vi "DisplayImagePlot.vi"(7 "Data Array":dbl[][](array[numeric]), 8 "Picture For Size Ref":refnum<vi>, 9 "Colormap":bool, 10 "Axis":bool, 11 "Map":T1) -> (2 "Picture":picture)   [LabVIEW 2018]
uses:
  <vilib>/Heliosphere Research LLC/Advanced Plotting Toolkit/properties/Colormap_Map.ctl
  <vilib>/Heliosphere Research LLC/Advanced Plotting Toolkit/api_plotting/ArrayViewProperties.ctl
  <vilib>/Heliosphere Research LLC/Advanced Plotting Toolkit/properties/Colormap.ctl
  <vilib>/Heliosphere Research LLC/Advanced Plotting Toolkit/properties/Colormap_Scaling.ctl
  <vilib>/Heliosphere Research LLC/Advanced Plotting Toolkit/properties/Display.ctl
  <vilib>/Heliosphere Research LLC/Advanced Plotting Toolkit/api_core/NewPlotProperties.ctl
  <vilib>/Heliosphere Research LLC/Advanced Plotting Toolkit/typedefs/PlotColor.ctl
  <vilib>/Heliosphere Research LLC/Advanced Plotting Toolkit/Advanced Plotting Toolkit.lvlib
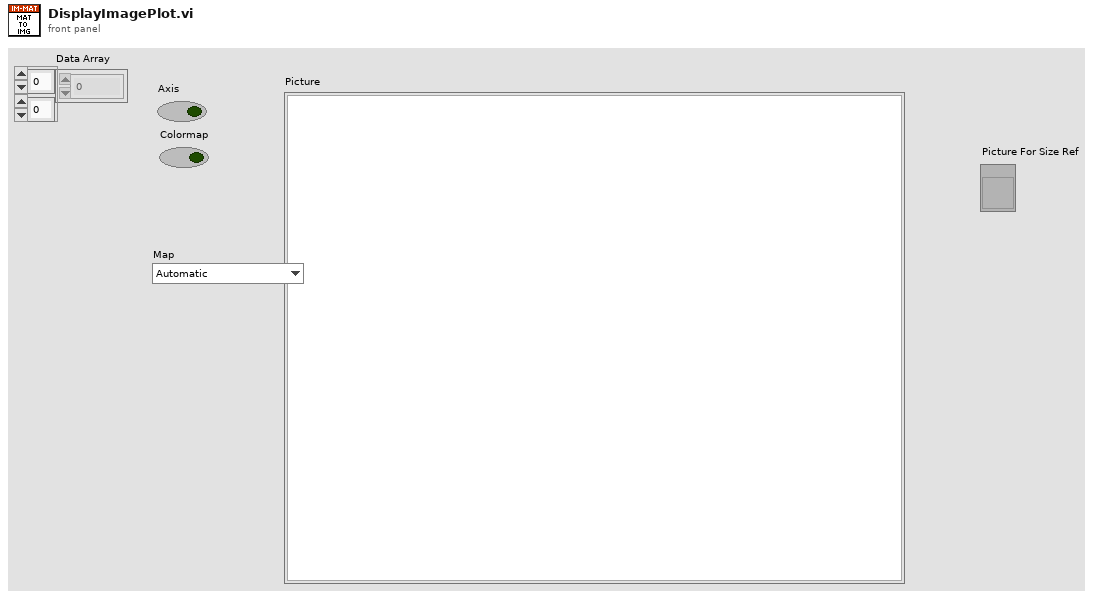
[diagram p1: front panel]
types:
  T1 = typedef "Advanced Plotting Toolkit.lvlib/Colormap_Map.ctl" = enum16{"Automatic", "Rainbow", "Hot and Cold", "White-Black", "White-Blue", "White-Green", "White-Red", "Fire", "Water", "Earth", "Air", "Pastel", "Banded", "Stepped"}
  T2 = typedef "Advanced Plotting Toolkit.lvlib/Colormap.ctl" = cluster{"Map":T1, "Value Min":dbl, "Value Max":dbl, "Scaling":T3, "Reverse":bool}
  T3 = typedef "Advanced Plotting Toolkit.lvlib/Colormap_Scaling.ctl" = enum16{"Default"}
  T4 = typedef "Advanced Plotting Toolkit.lvlib/ArrayViewProperties.ctl" = cluster{"Colormap":T2, "Display":T5}
  T5 = typedef "Advanced Plotting Toolkit.lvlib/Display.ctl" = cluster{"Alpha":dbl, "Z Order":dbl}
  T6 = typedef "Advanced Plotting Toolkit.lvlib/NewPlotProperties.ctl" = cluster{"Background Color":T7, "Axis Background":T7, "Left Margin":dbl, "Right Margin":dbl, "Bottom Margin":dbl, "Top Margin":dbl, "Aspect Ratio":dbl}
  T7 = typedef "Advanced Plotting Toolkit.lvlib/PlotColor.ctl" = u32
  T8 = typedef "Advanced Plotting Toolkit.lvlib/PlotID.ctl" = i32
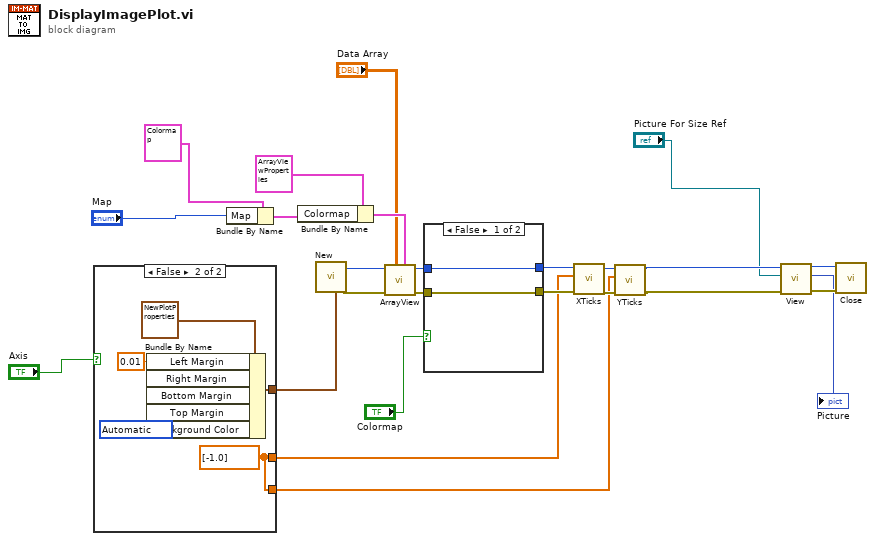
[diagram p0: block diagram]
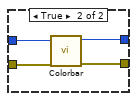
[diagram p2: hidden frame]
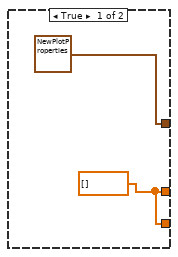
[diagram p3: hidden frame]
diagram:
  n1 = case shown="False" "Axis" {
    tunnel: [T6 {"Background Color"=2147483647, "Axis Background"=2147483647, "Left Margin"=nan, "Right Margin"=nan, "Bottom Margin"=nan, "Top Margin"=nan, "Aspect Ratio"=nan} ("Properties") w32] -> w20
    tunnel: [w26 w29] -> w14
    tunnel: [w26 w29] -> w15
    frame True {
      w26 = dbl[] [] ("Tick Locations")
    }
    frame False {
      w28 = T7 2147483647 items=["Automatic"=2147483647, "Black"=0, "White"=16777215, "Red"=16711680, "Green"=2263842, "Blue"=255, "Cyan"=65535, "Magenta"=16711935, "Yellow"=16776960] ("Axis Background")
      w29 = dbl[] [-1.0] ("Tick Locations")
      w30 = 0.01 ("Left Margin")
      n2 = Bundle By Name(cluster=T6 {"Background Color"=2147483647, "Axis Background"=2147483647, "Left Margin"=nan, "Right Margin"=nan, "Bottom Margin"=nan, "Top Margin"=nan, "Aspect Ratio"=nan} ("Properties"), "Left Margin"=w30, "Right Margin"=w30, "Bottom Margin"=w30, "Top Margin"=w30, "Background Color"=w28) -> (w32:T6)
    }
  }
  n3 = Bundle By Name(cluster=T2 {"Map"=enum."Automatic", "Value Min"=nan, "Value Max"=nan, "Scaling"=enum."Default", "Reverse"=FALSE} ("Colormap 2"), "Map"="Map") -> (w7:T2)
  n4 = Bundle By Name(cluster=T4 {"Colormap"={"Map"=enum."Automatic", "Value Min"=nan, "Value Max"=nan, "Scaling"=enum."Default", "Reverse"=FALSE}, "Display"={"Alpha"=nan, "Z Order"=nan}} ("Properties"), "Colormap"=w7) -> (w8:T4)
  n5 = call <vilib>:"New.vi"("Properties"=w20) -> ("error out"=w22:errorcluster, "Plot ID"=w23:T8)  [unwired: 9 in]
  n6 = call <vilib>:"ArrayView.vi"("Properties"=w8, "Data"="Data Array", "error in (no error)"=w22, "Plot ID"=w23) -> ("error out"=w25:errorcluster, "Plot ID Out"=w24:T8)  [unwired: 6 in]
  n7 = case shown="False" "Colormap" {
    tunnel: w25 -> [w33 w38]
    tunnel: w24 -> [w34 w37]
    tunnel: [w34 w36] -> w17
    tunnel: [w33 w35] -> w16
    frame False {
    }
    frame True {
      n8 = call <vilib>:"Colorbar.vi"("error in (no error)"=w38, "Plot ID"=w37) -> ("error out"=w35:errorcluster, "Plot ID Out"=w36:T8)  [unwired: 8 in]
    }
  }
  n9 = call <vilib>:"XTicks.vi"("error in (no error)"=w16, "Tick Locations"=w14, "Plot ID"=w17) -> ("error out"=w18:errorcluster, "Plot ID Out"=w19:T8)  [unwired: 7 in]
  n10 = call <vilib>:"YTicks.vi"("error in (no error)"=w18, "Tick Locations"=w15, "Plot ID"=w19) -> ("error out"=w3:errorcluster, "Plot ID Out"=w4:T8)  [unwired: 7 in]
  n11 = call <vilib>:"View.vi"("error in (no error)"=w3, "Ref for Sizing"="Picture For Size Ref", "Plot ID"=w4) -> ("error out"=w11:errorcluster, "Picture"=→"Picture":picture, "Plot ID Out"=w12:T8)  [unwired: 6 in]
  n12 = call <vilib>:"Close.vi"("error in (no error)"=w11, "Plot ID"=w12) -> ()  [unwired: 9 in, 1 out]
